vi "AO(Write).vi"() -> ()   [LabVIEW 2020]
uses:
  <instrlib>/HandsOnPi2040/Public/PWMSettings.ctl
  <instrlib>/HandsOnPi2040/Public/AOs.ctl
  <instrlib>/HandsOnPi2040/HandsOnPi2040.lvlib
panel:
  in  "stop":bool
  out "error out":errorcluster
  in  "Frequency":sgl(slide) scale=10.0..500000.0
  in  "Duty":sgl(slide) scale=0.0..1.0
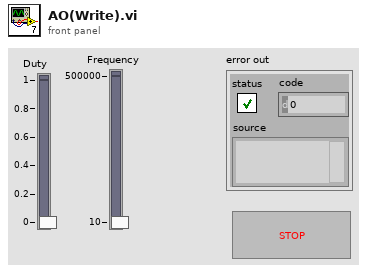
[diagram p1: front panel]
types:
  T1 = typedef "HandsOnPi2040.lvlib/AOs.ctl" = enum16{"No AO - Error", "AO1 (GPIO28)"}
  T2 = typedef "HandsOnPi2040.lvlib/PWMSettings.ctl" = cluster{"Duty":sgl, "Frequency":sgl}
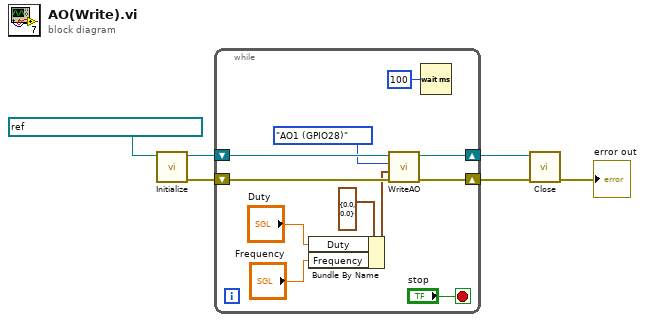
[diagram p0: block diagram]
diagram:
  n1 = call <instrlib>:"Initialize.vi"("VISA resource name"=refnum<visa-resource-name> "TCPIP0::10.0.2.15::6340::SOCKET") -> ("error out"=w3:errorcluster, "VISA resource name out"=w4:refnum<visa-resource-name>)  [unwired: 8 in, 1 out]
  n2 = while {
    shift-right: [w16] -> w5
    shift-left: w4 -> [w15]
    shift-right: [w17] -> w6
    shift-left: w3 -> [w14]
    stop <- "stop" stop-if-true
    n3 = Bundle By Name(cluster=T2 {"Duty"=0.0, "Frequency"=0.0} ("PWM Settings"), "Duty"="Duty", "Frequency"="Frequency") -> (w12:T2)
    n4 = call <instrlib>:"WriteAO.vi"("error in (no error)"=w14, "PWM Settings"=w12, "Analog Output"=AOs."AO1 (GPIO28)", "VISA resource name"=w15) -> ("error out"=w17:errorcluster, "VISA resource name out"=w16:refnum<visa-resource-name>)  [unwired: 6 in]
    n5 = Wait (ms)(milliseconds to wait=u32 100) -> ()  [unwired: 1 out]
  }
  n6 = call <instrlib>:"Close.vi"("error in (no error)"=w6, "VISA resource name"=w5) -> ("error out"=→"error out":errorcluster)  [unwired: 9 in]
